vi "Arm Hardware.vi"(8 "error in (no error)":errorcluster, 9 "Request type":T1=enum."User command", 11 "Micron sm Digitizer in":refnum<class "Micron sm Digitizer.lvclass">) -> (0 "error out":errorcluster, 3 "Micron sm Digitizer out":refnum<class "Micron sm Digitizer.lvclass">)   [LabVIEW 2024, in "Micron sm Digitizer.lvclass"]
uses:
  LabActor/Controllers/Process Controller/Request type.ctl
  Micron sm Digitizer.lvclass
  Micron sm Digitizer.lvclass/Micron sm Digitizer.ctl
  Micron Optics/Micron Optics Driver/Micron Optics Driver.lvclass
  Strain/Micron Optics sm130/Micron Optics sm130.lvlib
  File/File Class/File.lvclass
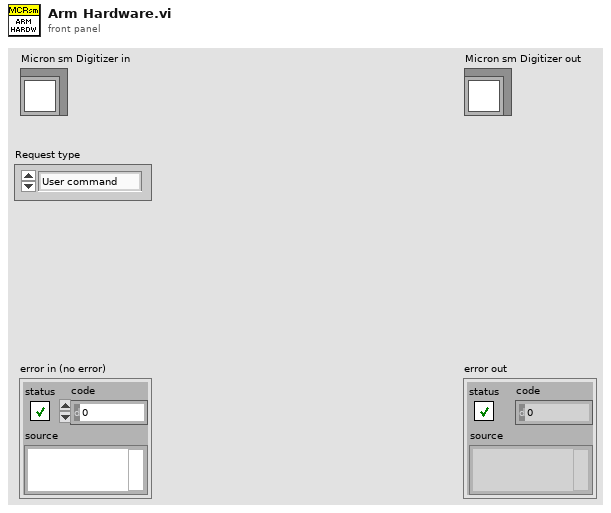
[diagram p1: front panel]
types:
  T1 = typedef "Request type.ctl" = enum16{"Process complete", "User command", "Auto-restart", "Error"}
  T2 = typedef "Micron optics didgitizer configuration.ctl" = cluster{"Post-trigger delay":dbl, "Post-trigger duration":dbl, "Rate":dbl, "Ranges":dbl[], "Re-name channels":string[], "Active channels":string, "External\nclock":bool, "Reference channel":i32, "Detection Setting IDs":u8[], "Stream and average":bool, "Address":string, "Number of sensors":i32}
  T3 = cluster{"Data Serial Number":u32, "Time Stamp":dbl, "Sub-Channel":u8}
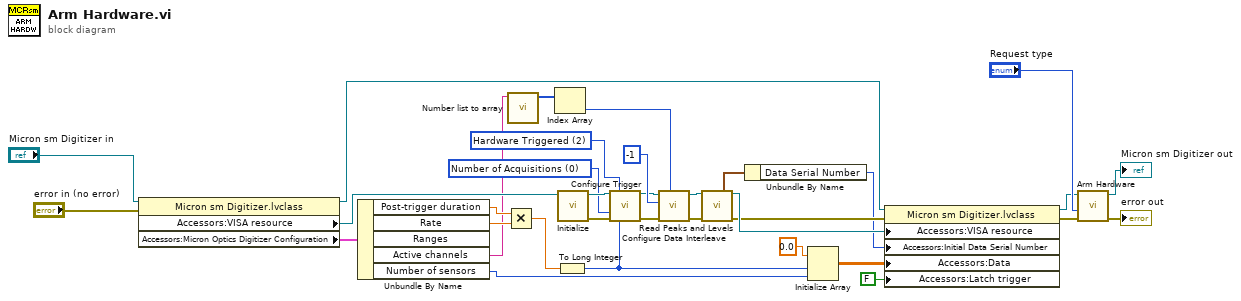
[diagram p0: block diagram]
diagram:
  w20 = u16 0 items=["Number of Acquisitions", "Edge Triggering"] ("Trigger Stop Condition (1:Edge Triggering)")
  w21 = u16 2 items=["Untriggered", "Software Triggered", "Hardware Triggered"] ("Trigger Type (0:Untriggered)")
  n1 = property class="Micron sm Digitizer.lvclass"(reference="Micron sm Digitizer in", error in="error in (no error)") -> (reference out=w13:refnum<class "Micron sm Digitizer.lvclass">, "Accessors:VISA resource"=w22:refnum<visa-resource-name>, "Accessors:Micron Optics Digitizer Configuration"=w19:T2)  [unwired: 1 out]
  n2 = Unbundle By Name(w19) -> ("Post-trigger duration"=w18:dbl, "Rate"=w17:dbl, "Active channels"=w8:string, "Number of sensors"=w4:i32)  [unwired: 1 out]
  n3 = Multiply(x=w18, y=w17) -> (x*y=w16:dbl)
  n4 = call "Number list to array.vi"("Number list"=w8) -> ("Number list array"=w7:i32[])  [unwired: 7 in, 3 out]
  n5 = Index Array(array=w7) -> (element=w6:i32)  [unwired: 1 in]
  n6 = To Long Integer(number=w16) -> (32bit integer=w3:i32)
  n7 = call "Initialize.vi"("VISA resource name"=w22) -> ("error out"=w26:errorcluster, "VISA resource name out"=w25:refnum<visa-resource-name>)  [unwired: 9 in]
  n8 = call "Configure Trigger.vi"("VISA resource name"=w25, "Trigger Type (0:Untriggered)"=w21, "Trigger Stop Condition (1:Edge Triggering)"=w20, "error in (no error)"=w26, "Number of Acquisitions (100)"=w3) -> ("VISA resource name out"=w23:refnum<visa-resource-name>, "error out"=w24:errorcluster)  [unwired: 8 in, 1 out]
  n9 = call "Configure Data Interleave.vi"("Channel (1: Channel 1)"=w6, "error in (no error)"=w24, "Sensor Number (1)"=-1, "VISA resource name"=w23) -> ("error out"=w28:errorcluster, "VISA resource name out"=w29:refnum<visa-resource-name>)  [unwired: 6 in]
  n10 = call "Read Peaks and Levels.vi"("VISA resource name"=w29, "error in (no error)"=w28) -> ("Data Status"=w15:T3, "VISA resource name out"=w12:refnum<visa-resource-name>, "error out"=w11:errorcluster)  [unwired: 5 in, 6 out]
  n11 = Unbundle By Name(w15) -> ("Data Serial Number"=w10:u32)
  n12 = Initialize Array(0.0 ("element"), w3, w4) -> (w2:dbl[][])
  n13 = property class="Micron sm Digitizer.lvclass"(reference=w13, error in=w11, "Accessors:VISA resource"=w12, "Accessors:Initial Data Serial Number"=w10, "Accessors:Data"=w2, "Accessors:Latch trigger"=FALSE ("Latch trigger")) -> (reference out=w14:refnum<class "Micron sm Digitizer.lvclass">, error out=w9:errorcluster)
  n14 = call-parent "Arm Hardware.vi"("error in (no error)"=w9, "Request type"="Request type", "Pulse Driver in"=w14) -> ("error out"=→"error out":errorcluster, "Pulse Driver out"=→"Micron sm Digitizer out":refnum<class "Micron sm Digitizer.lvclass">)  [unwired: 7 in]
